vi "SetOperationCycleStatus.vi"(8 "error in":errorcluster, 10 "OperationStatus":T1=enum."NOT_COMPLETED", 11 "OperationCycle in":refnum<class "OperationCycle.lvclass">) -> (0 "error out":errorcluster, 3 "OperationCycle out":refnum<class "OperationCycle.lvclass">)   [LabVIEW 2021, in "ProligentXMLGenerator.lvlib" / "OperationCycle.lvclass"]
doc: "Defines the last known status of the operation cycle.\nThis attribute can only be updated when closing the operation cycle (i.e. when providing a value for 'OperationCycleEndTime')."
uses:
  OperationCycle.lvclass
  OperationCycle.lvclass/OperationCycle.ctl
  Base/ExecutionStatus/Value.ctl
  Base/ExecutionStatus/ExecutionStatus.lvclass
  Base/DateTime/DateTime.lvclass
  Base/Attribute/Attribute.lvclass
  C:/Projects/proligent-xml-generator-labview/src/ProligentXMLGenerator/Base/Attribute/Attribute.lvclass
  C:/Projects/proligent-xml-generator-labview/src/ProligentXMLGenerator/Base/DateTime/DateTime.lvclass
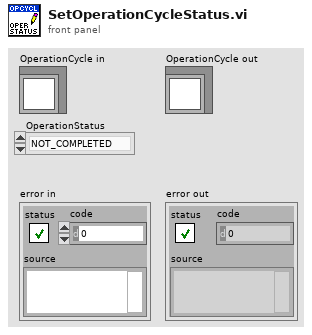
[diagram p1: front panel]
types:
  T1 = typedef "ProligentXMLGenerator.lvlib/ExecutionStatus.lvclass/Value.ctl" = enum16{"PASS", "FAIL", "NOT_COMPLETED", "ABORTED"}
  T2 = typedef "ProligentXMLGenerator.lvlib/OperationCycle.lvclass/Data.ctl" = cluster{"Name":string, "CustomData":refnum<class "CustomData.lvclass">, "ProcessFullName":refnum<class "ProcessFullName.lvclass">, "ProcessVersion":refnum<class "NonEmptyString_64.lvclass">, "OperationCycleId":refnum<class "Guid.lvclass">, "OperationName":refnum<class "NonEmptyString_65.lvclass">, "Location":refnum<class "FullName.lvclass">, "User":refnum<class "NonEmptyString_255.lvclass">, "OperationCycleStatus":refnum<class "ExecutionStatus.lvclass">, "OperationCycleStartTime":refnum<class "DateTime.lvclass">, "OperationCycleEndTime":refnum<class "DateTime.lvclass">, "TimeZoneInfoId":string}
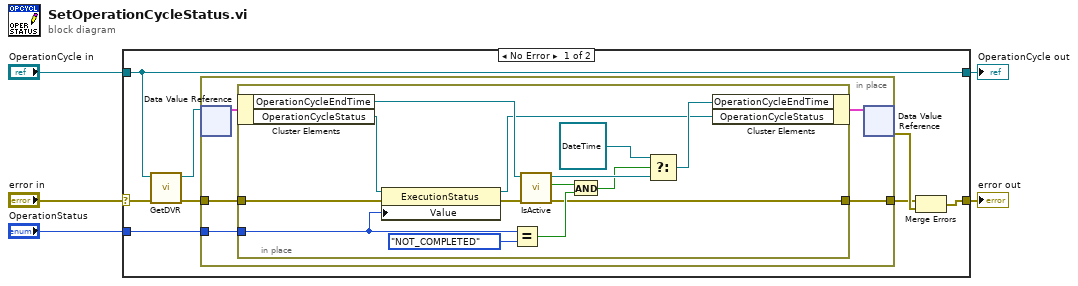
[diagram p0: block diagram]
diagram:
  n1 = case shown="No Error" "error in" {
    selector: "error in" -> [w11 w33]
    tunnel: "OperationCycle in" -> [w6 w34]
    tunnel: [w8 w33] -> w3
    tunnel: "OperationStatus" -> [w7 _]
    tunnel: [w6 w34] -> w1
    frame No Error {
      n2 = call "GetDVR.vi"("error in"=w11, "OperationCycle in"=w6) -> ("error out"=w10:errorcluster, "DVRReference"=w12:refnum<data-value>)  [unwired: 8 in]
      n3 = in-place "In Place Element Structure" {
        in-place-border: w10 -> [w18]
        in-place-border: [w16] -> w9
        in-place-border: w7 -> [w17]
        n4 = in-place-dvr #1(w12) -> (w15:T2)  [unwired: 1 out]
        n5 = in-place "In Place Element Structure" {
          in-place-border: w18 -> [w32]
          in-place-border: w17 -> [w31]
          in-place-border: [w26] -> w16
          n6 = in-place-cluster #2(w15) -> ("OperationCycleEndTime"=w22:refnum<class "DateTime.lvclass">, "OperationCycleStatus"=w21:refnum<class "ExecutionStatus.lvclass">)
          n7 = property on="Property Node" class="ExecutionStatus"(reference=w21, error in=w32, "Value"=w31) -> (reference out=w19:refnum<class "ExecutionStatus.lvclass">, error out=w29:errorcluster)
          n8 = Equal?(x=w31, y=Value."NOT_COMPLETED") -> (x = y?=w27:bool)
          n9 = call "IsActive.vi"("error in"=w29, "Attribute in"=w22) -> ("error out"=w26:errorcluster, "IsActive"=w28:bool, "Attribute in"=w24:refnum<class "DateTime.lvclass">)  [unwired: 7 in]
          n10 = And(x=w28, y=w27) -> (x .and. y?=w23:bool)
          n11 = Select(t=refnum<class "DateTime.lvclass"> refnum ("OperationRunEndTime"), s=w23, f=w24) -> (s? t:f=w20:refnum<class "DateTime.lvclass">)
          n12 = in-place-cluster #2("OperationCycleEndTime"=w20, "OperationCycleStatus"=w19) -> (w14:T2)
        }
        n13 = in-place-dvr #1(w14) -> (w13:errorcluster)  [unwired: 1 out]
      }
      n14 = Merge Errors(w9, w13) -> (w8:errorcluster)
    }
    frame Error {
    }
  }
  "error out" <- w3
  "OperationCycle out" <- w1
